vi "SetUp_Action.vi"(7 "Slot":T3, 8 "error in":errorcluster, 11 "GuiRef":T1={"StringOut"=refnum, "AbortOnFail"=refnum, "SN"=refnum, "SN_Length"=refnum, "TestResult"=refnum, "CycleTime"=refnum, "ErrorCode"=refnum, "UUTStatus"=refnum, "DataBaseEnable?"=refnum, "DUTModel"=refnum, "FixtureID"=refnum, "OperatorID"=refnum, "SNReady"=refnum, "StopSlot"=refnum, "NextStep"=refnum, "PassYeild"=refnum, "Failed"=refnum, "Passed"=refnum, "Tested"=refnum, "TestItemsCtl"={"StepName"="", "TestEnable"=FALSE, "LoopCount"=0, "StopOnFail"=FALSE, "Index"=0, "TestName"="", "通道"="", "参数"="", "TimeStart"=0}, "ProcessBar"=refnum, "Slot"=enum."Slot1", "Row"=3, "States"=refnum, "TestMode"=refnum, "循环次数-DUT"=refnum, "波形图"=refnum, "产品型号"=refnum, "子面板"=refnum, "测试失败项目"=refnum, "测试结果"=refnum, "DUT"=refnum, "Starttime"=refnum, "SlotReady"=refnum, "版本信息"=refnum}) -> (0 "error out":errorcluster, 3 "ScanSNOK":bool)   [LabVIEW 2013]
uses:
  SystemCode/SysControl/Slot.ctl
  SystemCode/SysControl/Reference.ctl
  SystemCode/SysControl/TestItemsCTL.ctl
  GlobalValue.vi
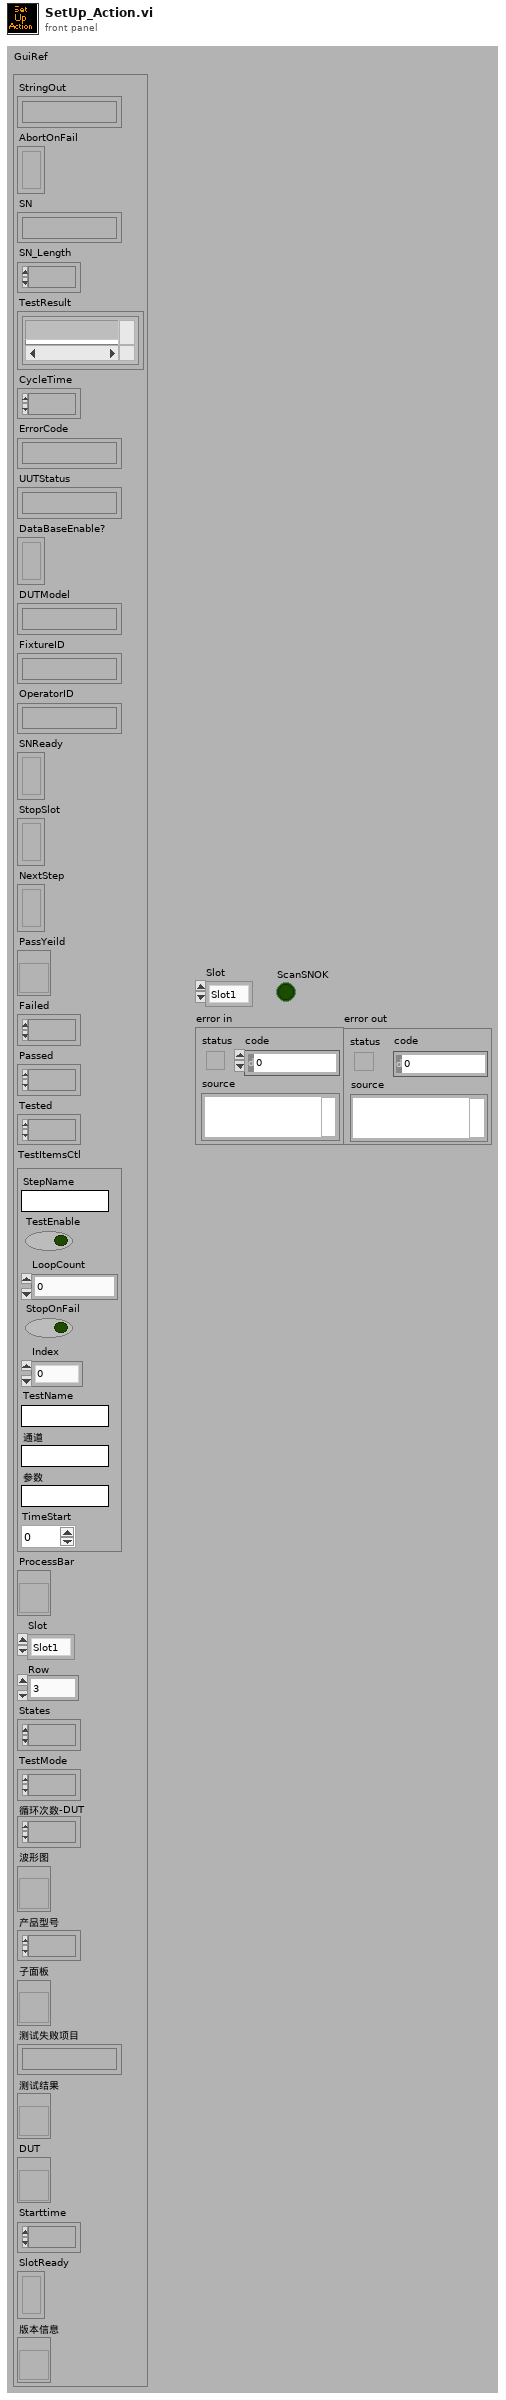
[diagram p1: front panel]
types:
  T1 = typedef "Reference.ctl" = cluster{"StringOut":refnum<vi>, "AbortOnFail":refnum<vi>, "SN":refnum<vi>, "SN_Length":refnum<vi>, "TestResult":refnum<vi>, "CycleTime":refnum<vi>, "ErrorCode":refnum<vi>, "UUTStatus":refnum<vi>, "DataBaseEnable?":refnum<vi>, "DUTModel":refnum<vi>, "FixtureID":refnum<vi>, "OperatorID":refnum<vi>, "SNReady":refnum<vi>, "StopSlot":refnum<vi>, "NextStep":refnum<vi>, "PassYeild":refnum<vi>, "Failed":refnum<vi>, "Passed":refnum<vi>, "Tested":refnum<vi>, "TestItemsCtl":T2, "ProcessBar":refnum<vi>, "Slot":T3, "Row":u32, "States":refnum<vi>, "TestMode":refnum<vi>, "循环次数-DUT":refnum<vi>, "波形图":refnum<vi>, "产品型号":refnum<vi>, "子面板":refnum<vi>, "测试失败项目":refnum<vi>, "测试结果":refnum<vi>, "DUT":refnum<vi>, "Starttime":refnum<vi>, "SlotReady":refnum<vi>, "版本信息":refnum<vi>}
  T2 = typedef "TestItemsCTL.ctl" = cluster{"StepName":string, "TestEnable":bool, "LoopCount":i32, "StopOnFail":bool, "Index":u32, "TestName":string, "通道":string, "参数":string, "TimeStart":u32}
  T3 = typedef "Slot.ctl" = enum16{"Slot1", "Slot2", "Slot3", "Slot4"}
  T4 = cluster{"InstrumentName":string, "VISA session":refnum<visa-resource-name>}[]
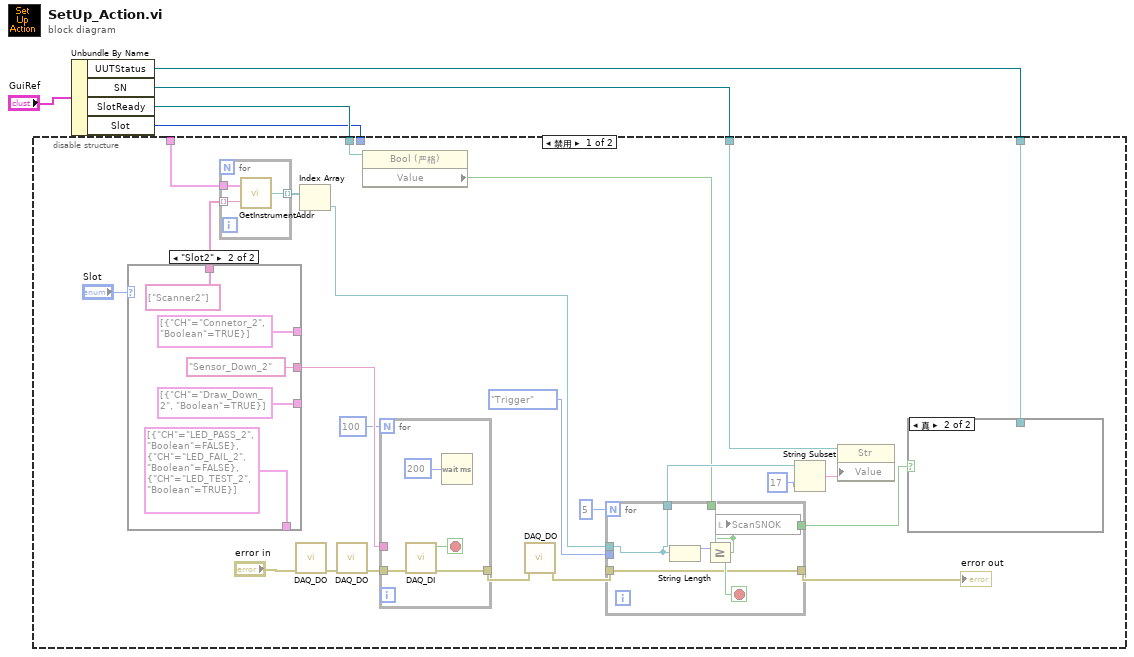
[diagram p0: block diagram]
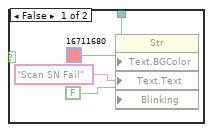
[diagram p2: hidden frame]
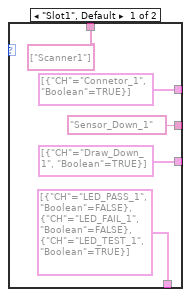
[diagram p3: hidden frame]
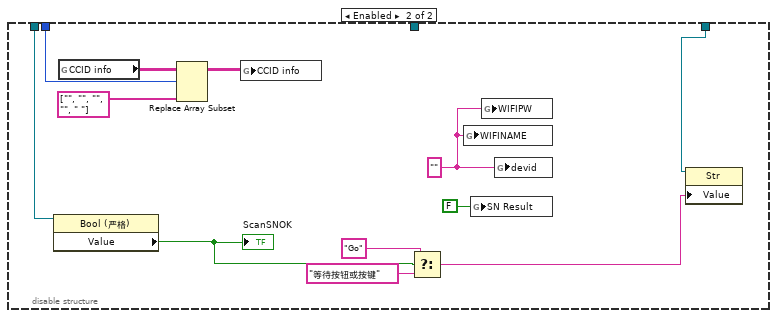
[diagram p4: hidden frame]
diagram:
  n1 = Unbundle By Name("GuiRef") -> ("UUTStatus"=w2:refnum<vi>, "SN"=w4:refnum<vi>, "SlotReady"=w3:refnum<vi>, "Slot"=w1:T3)
  n2 = disable-structure shown="禁用" {
    disable-tunnel: [w18 _] -> _
    disable-tunnel: w4 -> [w12 _]
    disable-tunnel: w3 -> [w9 w66]
    disable-tunnel: w2 -> [w6 w65]
    disable-tunnel: w1 -> [_ w59]
    frame Disabled {
      n3 = case shown="\"Slot2\"" "Slot" {
        tunnel: [cluster{"CH":string, "Boolean":bool}[] [{"CH"="Draw_Down_1", "Boolean"=TRUE}] ("Setting") cluster{"CH":string, "Boolean":bool}[] [{"CH"="Draw_Down_2", "Boolean"=TRUE}] ("Setting")] -> _
        tunnel: ["Sensor_Down_1" ("DILine") "Sensor_Down_2" ("DILine")] -> w26
        tunnel: [cluster{"CH":string, "Boolean":bool}[] [{"CH"="Connetor_1", "Boolean"=TRUE}] ("Setting") cluster{"CH":string, "Boolean":bool}[] [{"CH"="Connetor_2", "Boolean"=TRUE}] ("Setting")] -> _
        tunnel: [cluster{"CH":string, "Boolean":bool}[] [{"CH"="LED_PASS_1", "Boolean"=FALSE}, {"CH"="LED_FAIL_1", "Boolean"=FALSE}, {"CH"="LED_TEST_1", "Boolean"=TRUE}] ("Setting") cluster{"CH":string, "Boolean":bool}[] [{"CH"="LED_PASS_2", "Boolean"=FALSE}, {"CH"="LED_FAIL_2", "Boolean"=FALSE}, {"CH"="LED_TEST_2", "Boolean"=TRUE}] ("Setting")] -> _
        tunnel: [string[] ["Scanner1"] string[] ["Scanner2"]] -> w17
        frame "Slot1", Default {
        }
        frame "Slot2" {
        }
      }
      n4 = for {
        tunnel: [w40] -> w18
        tunnel: w17 -> [w39] mode=indexing
        tunnel: [w38] -> w16 mode=indexing
        n5 = call "GetInstrumentAddr.vi"("String"=w39) -> ("VISA session"=w38:refnum<visa-resource-name>, "Instruments"=w40:T4)
      }
      n6 = call "DAQ_DO.vi"("error in"="error in") -> ("error out"=w20:errorcluster)  [unwired: 10 in]
      n7 = Index Array(array=w16) -> (element=w15:refnum<visa-resource-name>)  [unwired: 1 in]
      n8 = call "DAQ_DO.vi"("error in"=w20) -> ("error out"=w25:errorcluster)  [unwired: 10 in]
      n9 = property class="Bool (严格)"(reference=w9) -> ("Value"=w8:bool)  [unwired: 1 in, 2 out]
      n10 = for {
        N: 100 -> [_]
        tunnel: w25 -> [w54]
        tunnel: w26 -> [_]
        tunnel: [w52] -> w21
        stop <- w53 stop-if-true
        n11 = call "DAQ_DI.vi"("error in"=w54) -> ("error out"=w52:errorcluster, "Status"=w53:bool)  [unwired: 9 in]
        n12 = Wait (ms)(milliseconds to wait=u32 200 ("等待时间（毫秒）")) -> ()  [unwired: 1 out]
      }
      n13 = call "DAQ_DO.vi"("error in"=w21) -> ("error out"=w22:errorcluster)  [unwired: 10 in]
      n14 = for {
        N: 5 -> [_]
        tunnel: enum16{"Trigger", "SetTriggerType"}."Trigger" ("Action") -> [_]
        tunnel: [w33] -> w24
        tunnel: w22 -> [w33]
        tunnel: w15 -> [w34]
        tunnel: [w34] -> w14
        tunnel: w8 -> [w36]
        tunnel: [w35] -> w7
        stop <- w35 stop-if-true
        n15 = String Length(string=w34) -> (length=w37:i32)
        n16 = Greater Or Equal?(x=w37, y=w36) -> (x >= y?=w35:bool)
        n17 = local write "ScanSNOK"(w35) -> ()
      }
      "error out" <- w24
      n18 = String Subset(string=w14, length (rest)=17 ("offset (0)")) -> (substring=w11:string)  [unwired: 1 in]
      n19 = property class="Str"(reference=w12, "Value"=w11) -> ()  [unwired: 1 in, 2 out]
      n20 = case shown="真" w7 {
        tunnel: w6 -> [w32 _]
        frame False {
          n21 = property on="Property Node" class="Str"(reference=w32, "Text.BGColor"=u32 16711680 ("Color Box 2"), "Text.Text"="Scan SN Fail", "Blinking"=FALSE) -> ()  [unwired: 1 in, 2 out]
        }
        frame True {
        }
      }
    }
    frame Enabled {
      w55 = "" ("devid")
      n22 = property class="Bool (严格)"(reference=w66) -> ("Value"=w64:bool)  [unwired: 1 in, 2 out]
      "ScanSNOK" <- w64
      n23 = global read "GlobalValue.vi" "CCID info"() -> (w60:string[][])
      n24 = Replace Array Subset(array=w60, new element=string[] ["", "", "", "", " "], index (row)=w59) -> (w57:string[][])  [unwired: 1 in]
      n25 = global write "GlobalValue.vi" "CCID info"(w57) -> ()
      n26 = Select(t="Go", s=w64, f="等待按钮或按键") -> (s? t:f=w61:string)
      n27 = global write "GlobalValue.vi" "WIFINAME"(w55) -> ()
      n28 = global write "GlobalValue.vi" "SN Result"(FALSE ("SN Result")) -> ()
      n29 = global write "GlobalValue.vi" "WIFIPW"(w55) -> ()
      n30 = global write "GlobalValue.vi" "devid"(w55) -> ()
      n31 = property class="Str"(reference=w65, "Value"=w61) -> ()  [unwired: 1 in, 2 out]
    }
  }
